vi "Gandalf Drive.vi"(1 "Tolerance":dbl=2.5 format="%#_13g", 2 "Min. Power":dbl, 3 "Reset":bool) -> (0 "Motor Powers":cluster{"RMotor":dbl, "LMotor":dbl})   [LabVIEW 2014]
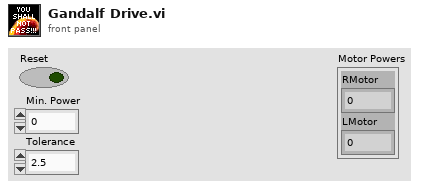
[diagram p1: front panel]
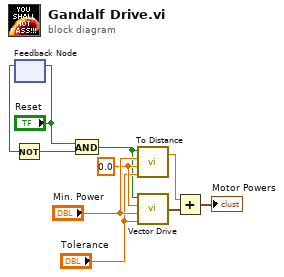
[diagram p0: block diagram]
diagram:
  w7 = 0.0 ("Angle")
  n1 = feedback-in #1("Reset") -> ()
  n2 = feedback #1() -> (w3:bool)  [unwired: 1 in]
  n3 = Not(x=w3) -> (.not. x?=w5:bool)
  n4 = And(x="Reset", y=w5) -> (x .and. y?=w2:bool)
  n5 = call "To Distance.vi"("Tolerance"="Tolerance", "Destination Dist (in)"=w7, "Min. Power"="Min. Power", "Reset"=w2) -> ("Base Speed"=w1:dbl)  [unwired: 1 out]
  n6 = call "Vector Drive.vi"("Tolerance"="Tolerance", "Min. Power"="Min. Power", "Angle"=w7, "Reset?"=w2) -> ("Motor Powers"=w9:cluster{"RMotor":dbl, "LMotor":dbl})
  n7 = Add(x=w1, y=w9) -> (x+y=→"Motor Powers":cluster{"RMotor":dbl, "LMotor":dbl})
